vi "Periodic Tasks.vi"(8 "error in":errorcluster, 11 "RobotConfig":T3={"Motors"={"DriveRightPrimary"={"CAN Address"=3, "Invert"=FALSE, "InvertSensor"=FALSE, "Unit Conversion Factor"=0.0, "Brake Mode"=enum."Override to Brake", "Reverse Limt Switch Mode"=enum."Normally Closed", "Forward Limt Swith Mode"=enum."Normally Closed", "PWM Channel"=enum."Invalid", "Motor Controller Type"=enum."Talon SRX"}, "DriveRightSecondary"={"CAN Address"=2, "Invert"=FALSE, "InvertSensor"=FALSE, "Unit Conversion Factor"=0.0, "Brake Mode"=enum."Override to Brake", "Reverse Limt Switch Mode"=enum."Normally Closed", "Forward Limt Swith Mode"=enum."Normally Closed", "PWM Channel"=enum."Invalid", "Motor Controller Type"=enum."Talon SRX"}, "DriveLeftPrimary"={"CAN Address"=1, "Invert"=FALSE, "InvertSensor"=FALSE, "Unit Conversion Factor"=0.0, "Brake Mode"=enum."Override to Brake", "Reverse Limt Switch Mode"=enum."Normally Closed", "Forward Limt Swith Mode"=enum."Normally Closed", "PWM Channel"=enum."Invalid", "Motor Controller Type"=enum."Talon SRX"}, "DriveLeftSecondary"={"CAN Address"=4, "Invert"=FALSE, "InvertSensor"=FALSE, "Unit Conversion Factor"=0.0, "Brake Mode"=enum."Override to Brake", "Reverse Limt Switch Mode"=enum."Normally Closed", "Forward Limt Swith Mode"=enum."Normally Closed", "PWM Channel"=enum."Invalid", "Motor Controller Type"=enum."Talon SRX"}, "RearClimb"={"CAN Address"=8, "Invert"=FALSE, "InvertSensor"=FALSE, "Unit Conversion Factor"=0.0, "Brake Mode"=enum."Override to Brake", "Reverse Limt Switch Mode"=enum."Normally Closed", "Forward Limt Swith Mode"=enum."Normally Closed", "PWM Channel"=enum."Invalid", "Motor Controller Type"=enum."Talon SRX"}, "Front Climb"={"CAN Address"=7, "Invert"=FALSE, "InvertSensor"=FALSE, "Unit Conversion Factor"=0.0, "Brake Mode"=enum."Override to Brake", "Reverse Limt Switch Mode"=enum."Normally Closed", "Forward Limt Swith Mode"=enum."Normally Closed", "PWM Channel"=enum."Invalid", "Motor Controller Type"=enum."Talon SRX"}, "Climb Drive"={"CAN Address"=5, "Invert"=FALSE, "InvertSensor"=FALSE, "Unit Conversion Factor"=0.0, "Brake Mode"=enum."Override to Brake", "Reverse Limt Switch Mode"=enum."Normally Closed", "Forward Limt Swith Mode"=enum."Normally Closed", "PWM Channel"=enum."Invalid", "Motor Controller Type"=enum."Talon SRX"}, "Shoulder1"={"CAN Address"=6, "Invert"=FALSE, "InvertSensor"=FALSE, "Unit Conversion Factor"=0.0, "Brake Mode"=enum."Override to Brake", "Reverse Limt Switch Mode"=enum."Normally Closed", "Forward Limt Swith Mode"=enum."Normally Closed", "PWM Channel"=enum."Invalid", "Motor Controller Type"=enum."Talon SRX"}, "Shoulder2"={"CAN Address"=9, "Invert"=FALSE, "InvertSensor"=FALSE, "Unit Conversion Factor"=0.0, "Brake Mode"=enum."Override to Brake", "Reverse Limt Switch Mode"=enum."Normally Closed", "Forward Limt Swith Mode"=enum."Normally Closed", "PWM Channel"=enum."Invalid", "Motor Controller Type"=enum."Talon SRX"}, "Wrist"={"CAN Address"=10, "Invert"=FALSE, "InvertSensor"=FALSE, "Unit Conversion Factor"=0.0, "Brake Mode"=enum."Override to Brake", "Reverse Limt Switch Mode"=enum."Disabled", "Forward Limt Swith Mode"=enum."Disabled", "PWM Channel"=enum."Invalid", "Motor Controller Type"=enum."Talon SRX"}, "Extension"={"CAN Address"=11, "Invert"=FALSE, "InvertSensor"=FALSE, "Unit Conversion Factor"=0.0, "Brake Mode"=enum."Override to Brake", "Reverse Limt Switch Mode"=enum."Disabled", "Forward Limt Swith Mode"=enum."Disabled", "PWM Channel"=enum."Invalid", "Motor Controller Type"=enum."Talon SRX"}, "Intake1"={"CAN Address"=11, "Invert"=FALSE, "InvertSensor"=FALSE, "Unit Conversion Factor"=0.0, "Brake Mode"=enum."Override to Brake", "Reverse Limt Switch Mode"=enum."Disabled", "Forward Limt Swith Mode"=enum."Disabled", "PWM Channel"=enum."Invalid", "Motor Controller Type"=enum."Talon SRX"}, "Intake2"={"CAN Address"=11, "Invert"=FALSE, "InvertSensor"=FALSE, "Unit Conversion Factor"=0.0, "Brake Mode"=enum."Override to Brake", "Reverse Limt Switch Mode"=enum."Disabled", "Forward Limt Swith Mode"=enum."Disabled", "PWM Channel"=enum."Invalid", "Motor Controller Type"=enum."Talon SRX"}}, "Sensors"={"IMU"={"Yaw Axis"=enum."Z", "SPI Bus"=enum."SPI MXP", "AHRS Algorithm"=enum."Complementary", "Calibration Time (s)"=3.0, "Calibrate On Open"=TRUE}}, "PID"={"PIDParams"={"P"=0.0, "I"=0.0, "D"=0.0, "F"=0.0, "IZone"=0.0}}, "Solenoids"={" Shifter"={"SolenoidChannel"=enum."Solenoid 3", "Invert"=FALSE}, "Intake 1"={"SolenoidChannel"=enum."Solenoid 0", "Invert"=FALSE}, "Intake 2"={"SolenoidChannel"=enum."Solenoid 0", "Invert"=FALSE}, "Claw"={"Forward Channel"=enum."Solenoid 0", "Invert"=FALSE, "Reverse Channel"=enum."Solenoid 0"}}, "Enable Compressor"=TRUE}) -> ()   [LabVIEW 2018]
doc: "This VI runs in parallel to other tasks. It can contain as many user-defined periodic loops as you need. These can carry out PID or other sorts of timed response."
uses:
  DeepSpaceSrc/TypeDefs/ConfigComponents/Config_Robot.ctl
  ArgosLib/Config/ConfigComponents/TypeDefs/Config_Motor.ctl
  <vilib>/Rock Robotics/WPI/ThirdParty/Phoenix-LabVIEW/Motor Controller/Controls/CTRE_Phoenix_MotorControl_NeutralMode.ctl
  <vilib>/Rock Robotics/WPI/ThirdParty/Phoenix-LabVIEW/Motor Controller/Controls/CTRE_Phoenix_MotorControl_LimitSwitchNormal.ctl
  <vilib>/Rock Robotics/SystemInterfaces/DIO/FPGA_DIOPWMChannel.ctl
  ArgosLib/Config/ConfigComponents/TypeDefs/Config_MotorCtrlType.ctl
  ArgosLib/Config/ConfigComponents/TypeDefs/Config_IMU.ctl
  <vilib>/Rock Robotics/SystemInterfaces/spilib/spi_bus.ctl
  ArgosLib/Config/ConfigComponents/TypeDefs/Config_PIDParams.ctl
  ArgosLib/Config/ConfigComponents/TypeDefs/Config_SingleSolenoid.ctl
  <vilib>/Rock Robotics/WPI/Solenoid/WPI_SolenoidChannel.ctl
  ArgosLib/Config/ConfigComponents/TypeDefs/Config_DoubleSolenoid.ctl
  ArgosLib/Miscellaneous/TypeDefs/ArgoDriveJoystickMap.ctl
  ArgosLib/Miscellaneous/TypeDefs/LookUpTableParameters.ctl
  <vilib>/Rock Robotics/WPI/Solenoid/WPI_SolenoidValue.ctl
  <vilib>/Rock Robotics/WPI/Utilities/WPI_GetSetVariantRefNum.vi
  DeepSpaceSrc/Global_Var-RefNum/Joystick_Control.vi
  <vilib>/Rock Robotics/WPI/Solenoid/WPI_SolenoidSetEnum.vi
  ArgosLib/ArgosLib.lvlib
panel:
  in  "Argo Drive Joystick Map":T1={"Auto Speed"={"Look Up Table OUT"=[-1.0, 0.0, 0.0, 0.0, 1.0], "Look Up Table IN"=[-1.0, -0.1, 0.0, 0.1, 1.0]}, "Low Speed"={"Look Up Table OUT"=[-1.0, 0.0, 0.0, 0.0, 1.0], "Look Up Table IN"=[-1.0, -0.1, 0.0, 0.1, 1.0]}, "Auto Turning"={"Look Up Table OUT"=[-1.0, -0.1, 0.0, 0.1, 1.0], "Look Up Table IN"=[-1.0, -0.1, 0.0, 0.1, 1.0]}, "Low Turning"={"Look Up Table OUT"=[-1.0, 0.0, 0.0, 0.0, 1.0], "Look Up Table IN"=[-1.0, -0.1, 0.0, 0.1, 1.0]}, "High Speed"={"Look Up Table OUT"=[-1.0, 0.0, 0.0, 0.0, 1.0], "Look Up Table IN"=[-1.0, -0.1, 0.0, 0.1, 1.0]}, "High Turning"={"Look Up Table OUT"=[-1.0, 0.0, 0.0, 0.0, 1.0], "Look Up Table IN"=[-1.0, -0.1, 0.0, 0.1, 1.0]}}
  out "LED Loop Rate (Hz)":dbl
  out "Implement Loop Rate (Hz)":dbl
  out "Compressor Loop Rate (Hz)":dbl
  out "Drive Loop Rate (Hz)":dbl
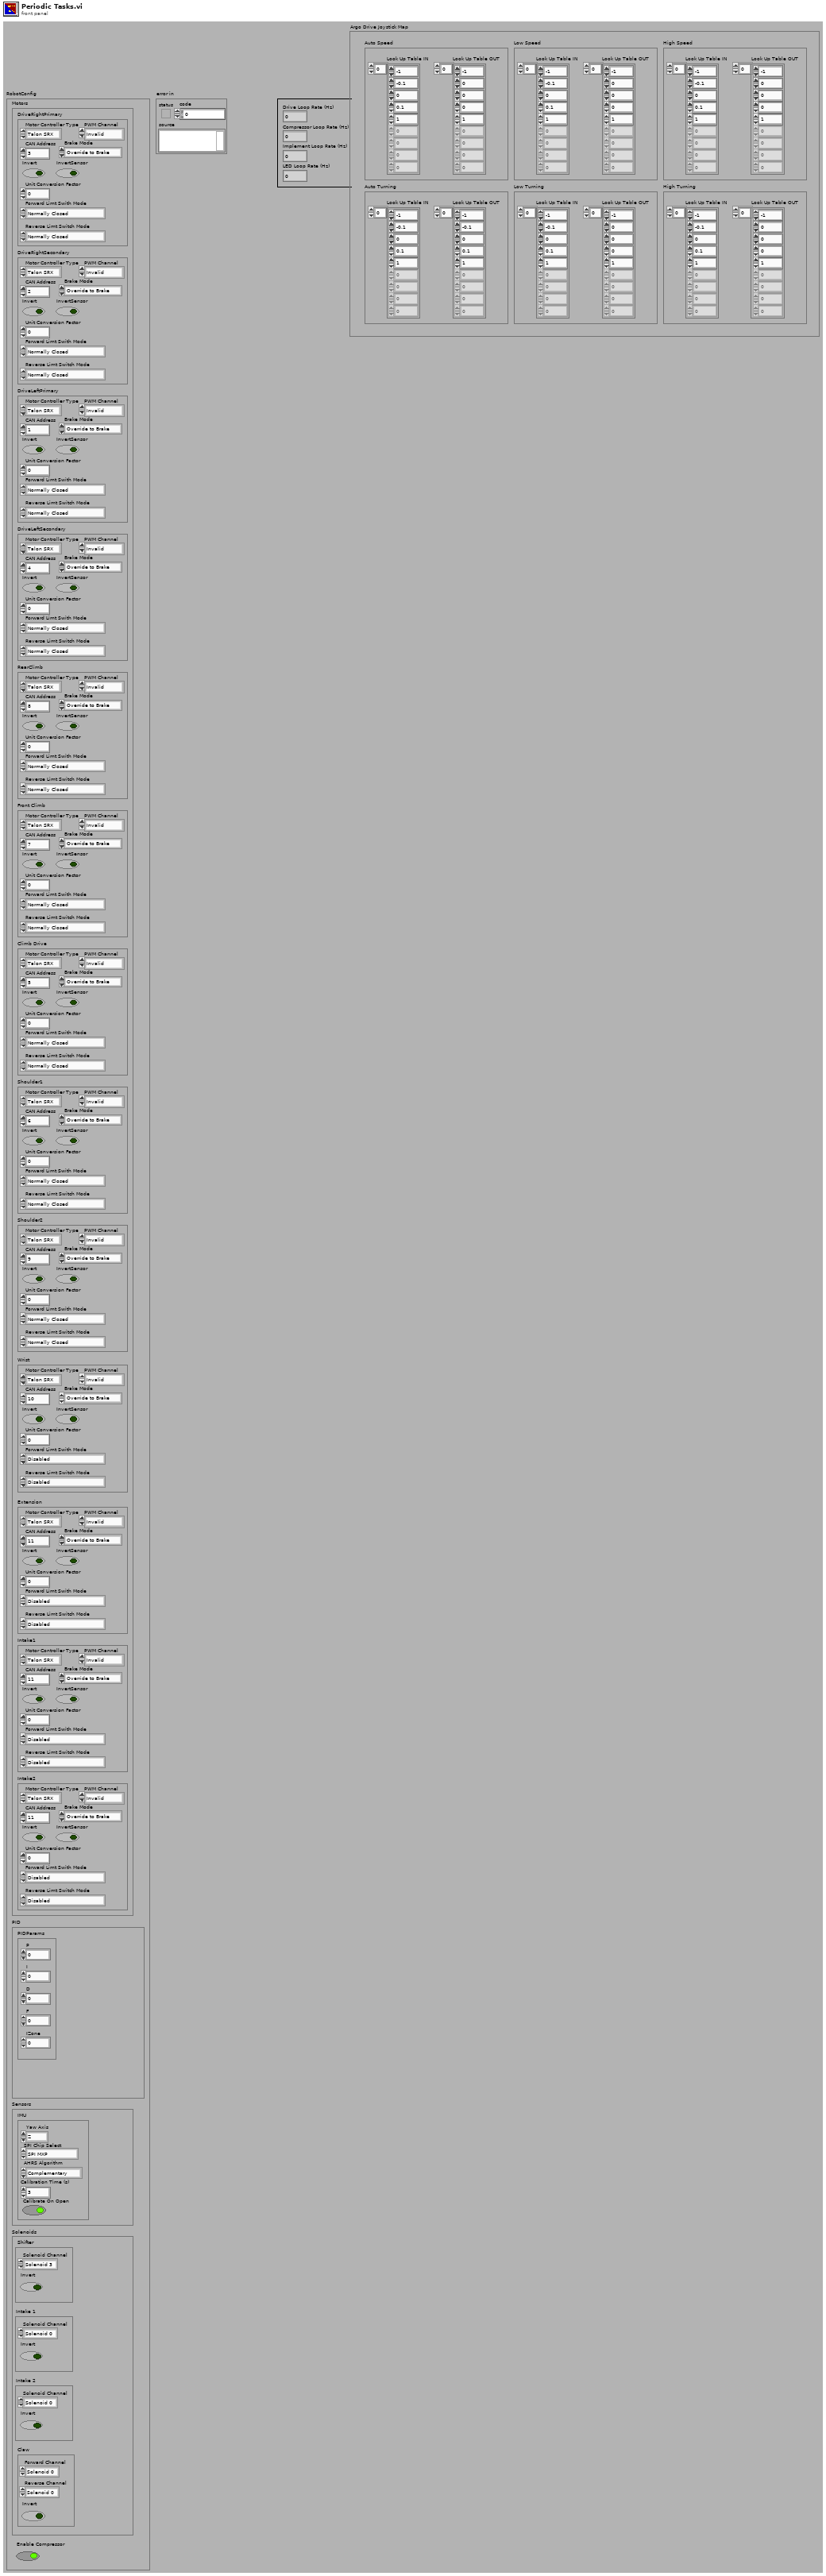
[diagram p1: front panel]
types:
  T1 = typedef "ArgosLib.lvlib/ArgoDriveJoystickMap.ctl" = cluster{"Auto Speed":T2, "Low Speed":T2, "Auto Turning":T2, "Low Turning":T2, "High Speed":T2, "High Turning":T2}
  T2 = typedef "ArgosLib.lvlib/LookUpTableParameters.ctl" = cluster{"Look Up Table OUT":dbl[], "Look Up Table IN":dbl[]}
  T3 = typedef "Config_Robot.ctl" = cluster{"Motors":cluster{"DriveRightPrimary":T4, "DriveRightSecondary":T4, "DriveLeftPrimary":T4, "DriveLeftSecondary":T4, "RearClimb":T4, "Front Climb":T4, "Climb Drive":T4, "Shoulder1":T4, "Shoulder2":T4, "Wrist":T4, "Extension":T4, "Intake1":T4, "Intake2":T4}, "Sensors":cluster{"IMU":T9}, "PID":cluster{"PIDParams":T11}, "Solenoids":cluster{" Shifter":T12, "Intake 1":T12, "Intake 2":T12, "Claw":T14}, "Enable Compressor":bool}
  T4 = typedef "ArgosLib.lvlib/Config_Motor.ctl" = cluster{"CAN Address":u8, "Invert":bool, "InvertSensor":bool, "Unit Conversion Factor":dbl, "Brake Mode":T5, "Reverse Limt Switch Mode":T6, "Forward Limt Swith Mode":T6, "PWM Channel":T7, "Motor Controller Type":T8}
  T5 = typedef "CTRE_Phoenix_MotorControl_NeutralMode.ctl" = enum8{"EEPROMSetting", "Override to Coast", "Override to Brake"}
  T6 = typedef "CTRE_Phoenix_MotorControl_LimitSwitchNormal.ctl" = enum16{"Normally Open", "Normally Closed", "Disabled"}
  T7 = typedef "FPGA_DIOPWMChannel.ctl" = enum8{"PWM 0", "PWM 1", "PWM 2", "PWM 3", "PWM 4", "PWM 5", "PWM 6", "PWM 7", "PWM 8", "PWM 9", "PWM MXP 0", "PWM MXP 1", "PWM MXP 2", "PWM MXP 3", "PWM MXP 4", "PWM MXP 5", "PWM MXP 6", "PWM MXP 7", "PWM MXP 8", "PWM MXP 9", "Invalid"}
  T8 = typedef "ArgosLib.lvlib/Config_MotorCtrlType.ctl" = enum16{"Disabled", "Talon SRX", "Talon SR"}
  T9 = typedef "ArgosLib.lvlib/Config_IMU.ctl" = cluster{"Yaw Axis":enum16{"X", "Y", "Z"}, "SPI Bus":T10, "AHRS Algorithm":enum16{"Complementary", "Madgwick"}, "Calibration Time (s)":dbl, "Calibrate On Open":bool}
  T10 = typedef "spi_bus.ctl" = enum16{"SPI On-Board, CS0", "SPI On-Board, CS1", "SPI On-Board, CS2", "SPI On-Board, CS3", "SPI MXP", "Invalid"}
  T11 = typedef "ArgosLib.lvlib/Config_PIDParams.ctl" = cluster{"P":dbl, "I":dbl, "D":dbl, "F":dbl, "IZone":dbl}
  T12 = typedef "ArgosLib.lvlib/Config_SingleSolenoid.ctl" = cluster{"SolenoidChannel":T13, "Invert":bool}
  T13 = typedef "WPI_SolenoidChannel.ctl" = enum8{"Solenoid 0", "Solenoid 1", "Solenoid 2", "Solenoid 3", "Solenoid 4", "Solenoid 5", "Solenoid 6", "Solenoid 7", "Invalid"}
  T14 = typedef "ArgosLib.lvlib/Config_DoubleSolenoid.ctl" = cluster{"Forward Channel":T13, "Invert":bool, "Reverse Channel":T13}
  T15 = typedef "RobotJoysticks.ctl" = cluster{"Driver Controller":T16, "Operator Controller":T16, "Manual Controller":T16}
  T16 = typedef "WPI_JoystickDevRef.ctl" = cluster{"Device":T17}
  T17 = typedef "WPI_JoystickDeviceEnum.ctl" = enum16{"USB 0", "USB 1", "USB 2", "USB 3", "USB 4", "USB 5"}
  T18 = typedef "WPI_RobotDriveDevRef.ctl" = cluster{"DevStatus":errorcluster, "Motors[]":T19[], "Square Inputs":bool, "Max Output":dbl}
  T19 = typedef "WPI_MotorControlDeviceRef.ctl" = cluster{"DeviceStatus":errorcluster, "Type":T20, "PWM":cluster{"PWM Channel":T7, "DeadBand":T21}, "CAN":cluster{"Device Number":u8, "SetOutput VI Ref":variant, "GetOutput VI Ref":variant, "Enable VI Ref":variant, "Disable VI Ref":variant, "Data":variant}, "Invert":bool, "DIO PWM":cluster{"PWM \"Enable\" Channel":T7, "DIOChannel":T22, "PWM Rate":dbl}}
  T20 = typedef "WPI_MotorControlType.ctl" = enum16{"PWM", "CAN", "DIO PWM"}
  T21 = typedef "WPI_PWMDeadband.ctl" = cluster{"Name":string, "maxPositivePwm":i32, "minPositivePwm":i32, "centerPwm":i32, "maxNegativePwm":i32, "minNegativePwm":i32, "angularRange":u16}
  T22 = typedef "FPGA_DIOChannel.ctl" = enum8{"DIO 0", "DIO 1", "DIO 2", "DIO 3", "DIO 4", "DIO 5", "DIO 6", "DIO 7", "DIO 8", "DIO 9", "DIO MXP 0", "DIO MXP 1", "DIO MXP 2", "DIO MXP 3", "DIO MXP 4", "DIO MXP 5", "DIO MXP 6", "DIO MXP 7", "DIO MXP 8", "DIO MXP 9", "DIO MXP 10", "DIO MXP 11", "DIO MXP 12", "DIO MXP 13", "DIO MXP 14", "DIO MXP 15", "SPI Port CS1", "SPI Port CS2", "SPI Port CS3", "SPI Port MISO", "SPI Port MOSI", "Invalid"}
  T23 = typedef "RobotMotors.ctl" = cluster{"DriveRightPrimary":T19, "DriveRightSecondary":T19, "DriveLeftPrimary":T19, "DriveLeftSecondary":T19, " RearClimb":T19, "FrontClimb":T19, "ClimbDrive":T19, "Shoulder2":T19, "Shoulder1 ":T19, "Wrist":T19, "Extension":T19, "Intake1":T19, "Intake2":T19}
  T24 = typedef "RobotPneumatics.ctl" = cluster{"Shifter":T25, "Compressor":T26, "Claw":T25, "Intake 1":T25, "Intake 2":T25}
  T25 = typedef "WPI_SolenoidDevRef.ctl" = cluster{"DevStatus":errorcluster, "Pneumatics Control Module":u8, "Forward Solenoid Channel":T13, "Reverse Solenoid Channel":T13}
  T26 = typedef "WPI_CompressorDevRef.ctl" = cluster{"DevStatus":errorcluster, "Pneumatics Control Module":u8}
  T27 = typedef "RobotSensors.ctl" = cluster{"DigitalIOConfig":T28}
  T28 = typedef "ArgosLib.lvlib/Config_DigitalIO.ctl" = cluster{"DIOChannel":T22, "Active Low":bool}
  T29 = cluster{"RobotConfig":T3, "Joysticks":T15, "RobotDriveDevRef":T18, "RobotMotorsOut":T23, "Pneumatics":T24, "Sensors":T27}
  T30 = typedef "WPI_SolenoidValue.ctl" = enum16{"Off", "On", "Forward", "Reverse"}
  T31 = typedef "JoystickControls.ctl" = cluster{"Drive":dbl, "Drive Turn ":dbl, "Unassigned_LX":dbl, "Unassigned_RY":dbl, "Claw Release":bool, "Back Intake Forward":dbl, "Front Intake Forward":dbl, "SP Low":bool, "SP Mid":bool, "SP High":bool, "Shift":bool, "Arm Go To Position":bool, "Unassigned_LJ":bool, "Unassigned_RJ":bool, "Swap_Back":bool, "Swap_Start":bool, "Unassigned_LY 2":dbl, "Unassigned_RX 2":dbl, "Unassigned_LX 2":dbl, "Unassigned_RY 2":dbl, "Claw Release 2":bool, "Back Intake REV":dbl, "Front Intake REV":dbl, "SP Low 2":bool, "SP Mid 2":bool, "SP High 2":bool, "Hatch/Cargo":bool, "Fwd/Rev":bool, "Unassigned_LJ 2":bool, "Unassigned_RJ 2":bool, "Swap_Back 2":bool, "Swap_Start 2":bool, "Unassigned_Up 2":bool, "Unassigned_Right 2":bool, "Arm Return":bool, "Unassigned_Left 2":bool, "Auto Climb":bool, " Unassigned_Right":bool, "Unassigned_Down":bool, "Unassigned_Left":bool, "Shoulder":dbl, "Unassigned_RX 3":dbl, "Unassigned_LX 3":dbl, "Arm Extend":dbl, "Climb Drive Reverse":bool, "Wrist CCW":dbl, "Wrist CW":dbl, "Rev Intake Extend":bool, "Fw Intake Extend":bool, "Climb Dr Forward":bool, "Intake Ingest ":bool, "Claw Release 3":bool, "Unassigned_LJ 3":bool, "Unassigned_RJ 3":bool, "Intake Puke":bool, "Unassigned Start 3":bool, "Climb F Up":bool, "Climb R Up":bool, "Climb F Down":bool, "Climb R Down":bool}
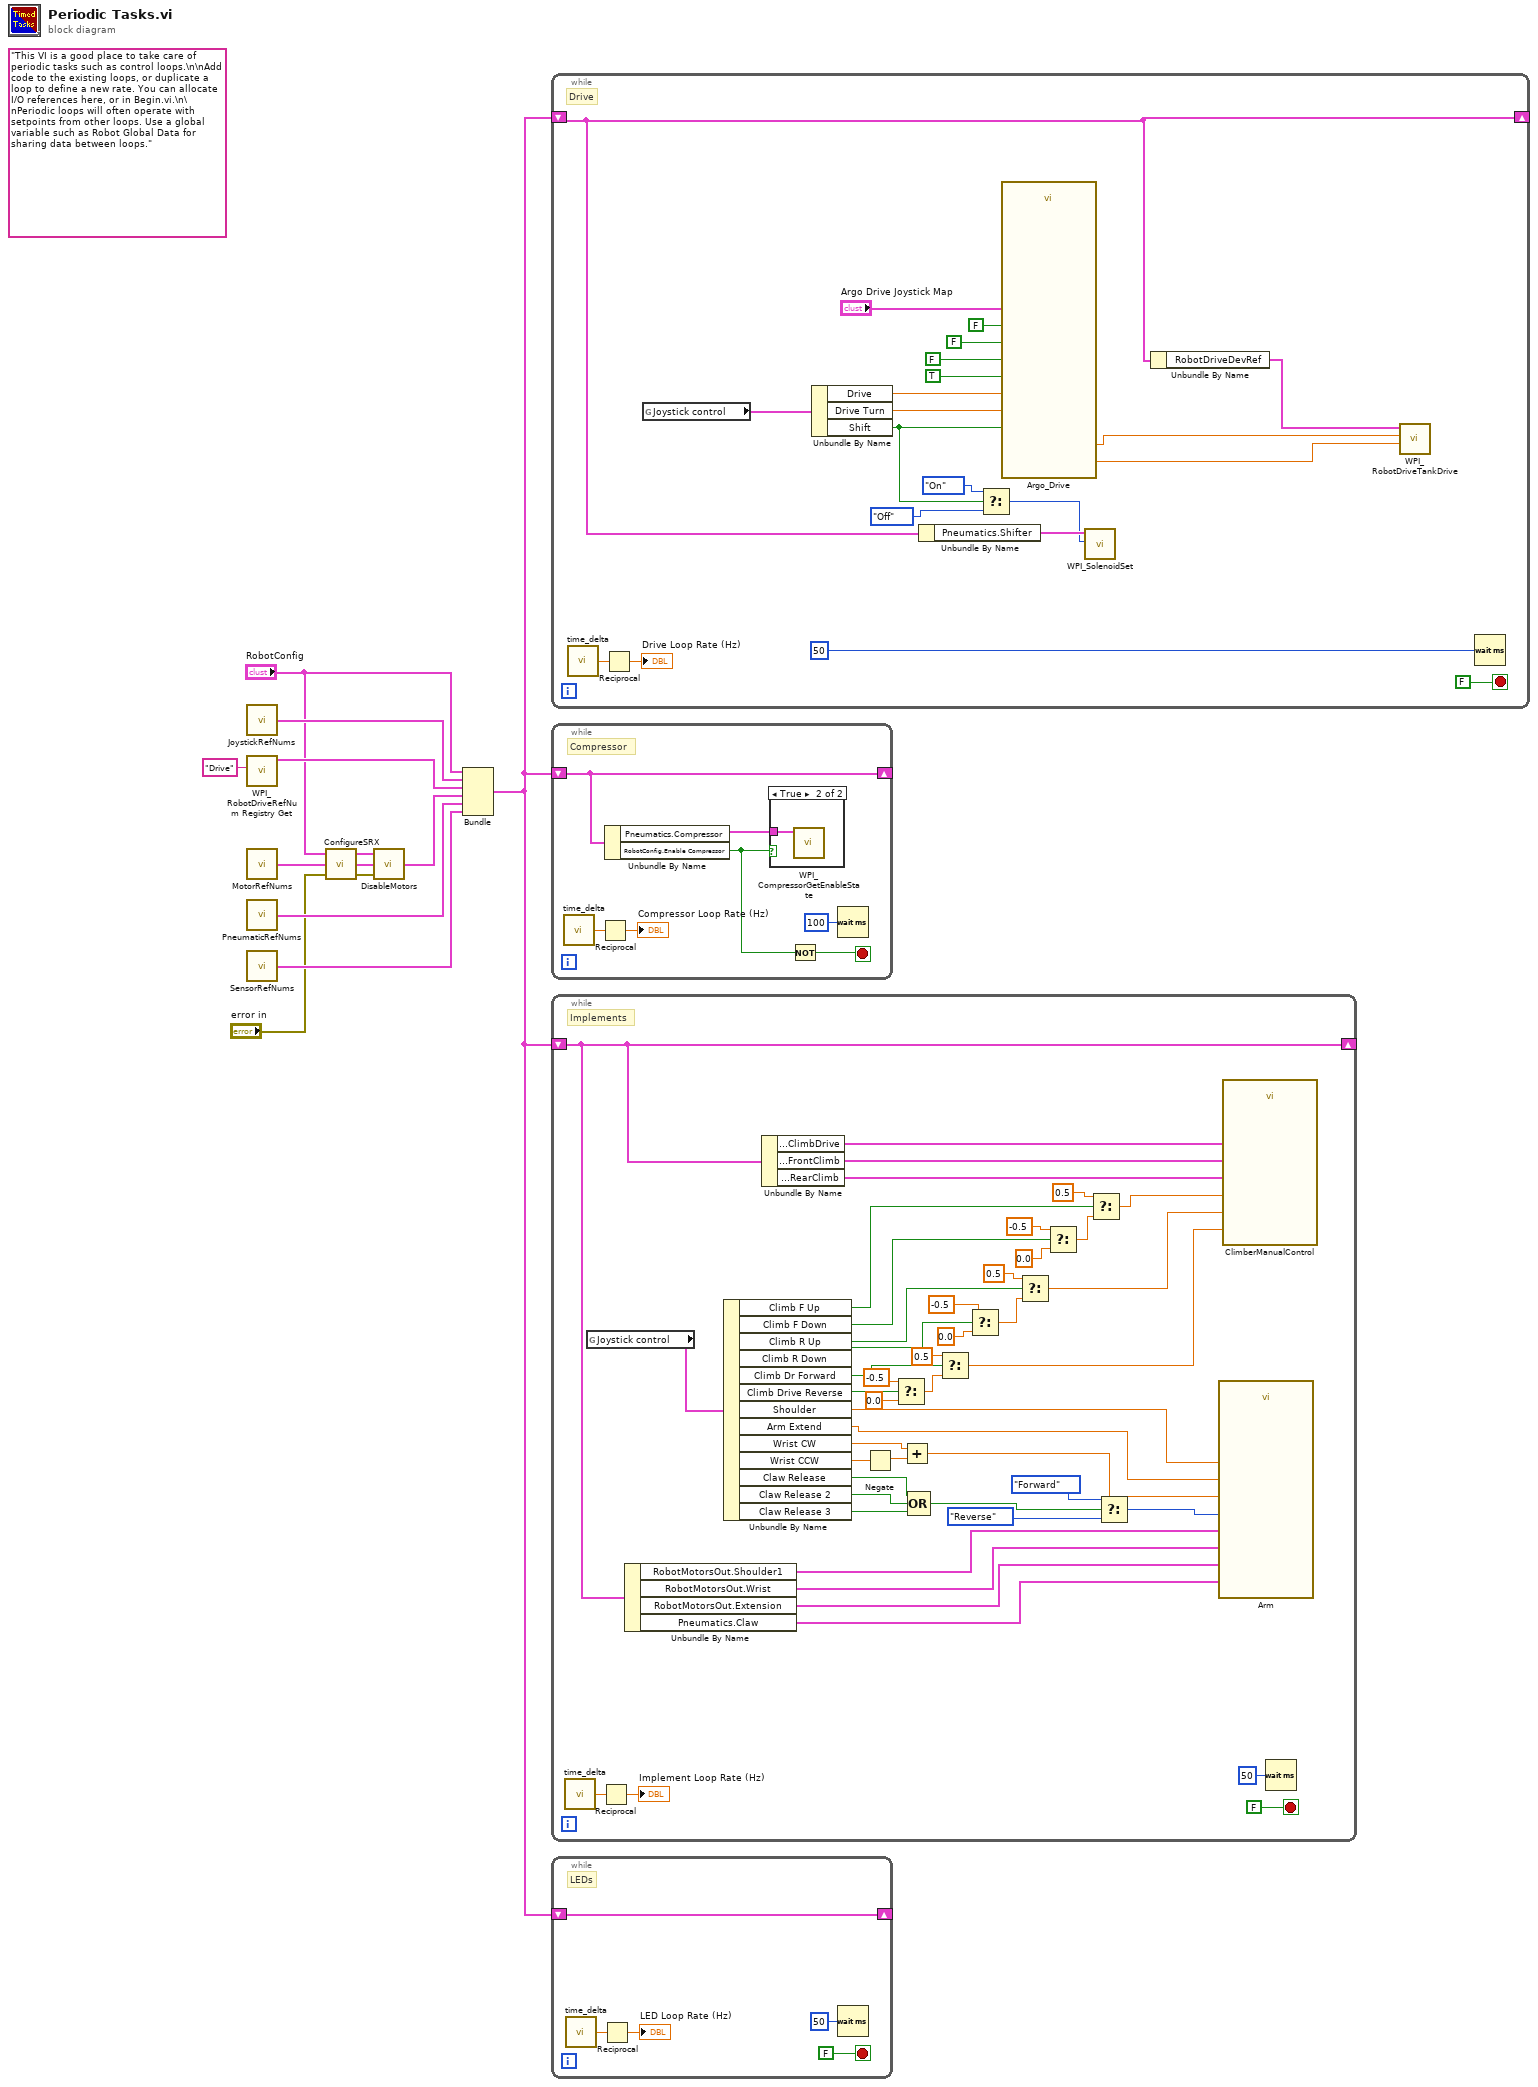
[diagram p0: block diagram]
diagram:
  (unwired) "This VI is a good place to take care of periodic tasks such as control loops.\n\nAdd code to the existing loops, or duplicate a loop to define a new rate. You can allocate I/O references here, or in Begin.vi.\n\nPeriodic loops will often operate with setpoints from other loops. Use a global variable such as Robot Global Data for sharing data between loops."
  n1 = call "JoystickRefNums.vi"() -> ("Joysticks"=w13:T15)  [unwired: 1 in]
  n2 = call <vilib>:"WPI_RobotDriveRefNum Registry Get.vi"("refnum name"="Drive") -> ("RobotDriveDevRef"=w12:T18)  [unwired: 9 in, 1 out]
  n3 = call "MotorRefNums.vi"() -> ("MotorRefNums"=w5:T23)  [unwired: 1 in]
  n4 = call "PneumaticRefNums.vi"() -> ("Pneumatics"=w11:T24)  [unwired: 1 in]
  n5 = call "SensorRefNums.vi"() -> ("Sensors"=w10:T27)  [unwired: 1 in]
  n6 = call "ConfigureSRX.vi"("error in"="error in", "RobotMotors"=w5, "RobotConfig"="RobotConfig") -> ("error out"=w9:errorcluster, "RobotMotorsOut"=w7:T23, "RobotConfigOut"=w8:T3)
  n7 = call "DisableMotors.vi"("error in"=w9, "RobotMotors"=w7, "RobotConfig"=w8) -> ("RobotMotorsOut"=w3:T23)  [unwired: 2 out]
  n8 = Bundle("RobotConfig"="RobotConfig", "Joysticks"=w13, "RobotDriveDevRef"=w12, "RobotMotorsOut"=w3, "Pneumatics"=w11, "Sensors"=w10) -> (w1:T29)  [unwired: 1 out]
  n9 = while {
    shift-right: [w19] -> _
    shift-left: w1 -> [w19]
    stop <- FALSE stop-if-true
    # "Drive"
    n10 = call "time_delta.vi"() -> ("dt (s)"=w32:dbl)  [unwired: 1 in]
    n11 = Reciprocal(x=w32) -> (1/x=→"Drive Loop Rate (Hz)":dbl)
    n12 = global read "Joystick_Control.vi" "Joystick control"() -> (w30:T31)
    n13 = Unbundle By Name(w30) -> ("Drive"=w28:dbl, "Drive Turn"=w29:dbl, "Shift"=w17:bool)
    n14 = Unbundle By Name(w19) -> ("Pneumatics.Shifter"=w18:T25)
    n15 = Select(t=WPI_SolenoidValue."On", s=w17, f=WPI_SolenoidValue."Off" ("Value")) -> (s? t:f=w15:T30)
    n16 = call "Argo_Drive.vi"("Speed_Main"=w28, "Argo Drive Joystick Map"="Argo Drive Joystick Map", "Backwards_Turning_Flip"=FALSE, "Turning_PID_Enable"=FALSE, "Turning_Main"=w29, "Auto_Enable"=FALSE, "High_Gear"=w17, "Quick_Turn"=TRUE) -> ("Left_Motor"=w22:dbl, "Right_Motor"=w21:dbl)  [unwired: 10 in]
    n17 = call-poly <vilib>:"WPI_SolenoidSet.vi"("Value"=w15, "SolenoidDevRef"=w18) -> ()  [unwired: 8 in, 2 out]
    n18 = Unbundle By Name(w19) -> ("RobotDriveDevRef"=w20:T18)
    n19 = call <vilib>:"WPI_RobotDriveTankDrive.vi"("Right axis value"=w21, "Left axis value"=w22, "RobotDriveDevRef"=w20) -> ()  [unwired: 6 in, 3 out]
    n20 = Wait (ms)(milliseconds to wait=u32 50) -> ()  [unwired: 1 out]
  }
  n21 = while {
    shift-right: [w38] -> _
    shift-left: w1 -> [w38]
    stop <- w37 stop-if-true
    # "Compressor"
    n22 = call "time_delta.vi"() -> ("dt (s)"=w39:dbl)  [unwired: 1 in]
    n23 = Reciprocal(x=w39) -> (1/x=→"Compressor Loop Rate (Hz)":dbl)
    n24 = Unbundle By Name(w38) -> ("Pneumatics.Compressor"=w35:T26, "RobotConfig.Enable Compressor"=w36:bool)
    n25 = case shown="True" w36 {
      tunnel: w35 -> [_ w42]
      frame False {
      }
      frame True {
        n26 = call <vilib>:"WPI_CompressorGetEnableState.vi"("CompressorDevRef"=w42) -> ()  [unwired: 7 in, 4 out]
      }
    }
    n27 = Not(x=w36) -> (.not. x?=w37:bool)
    n28 = Wait (ms)(milliseconds to wait=u32 100) -> ()  [unwired: 1 out]
  }
  n29 = while {
    shift-right: [w60] -> _
    shift-left: w1 -> [w60]
    stop <- FALSE stop-if-true
    # "Implements"
    n30 = call "time_delta.vi"() -> ("dt (s)"=w87:dbl)  [unwired: 1 in]
    n31 = global read "Joystick_Control.vi" "Joystick control"() -> (w85:T31)
    n32 = Reciprocal(x=w87) -> (1/x=→"Implement Loop Rate (Hz)":dbl)
    n33 = Unbundle By Name(w60) -> ("RobotMotorsOut.Shoulder1"=w59:T19, "RobotMotorsOut.Wrist"=w58:T19, "RobotMotorsOut.Extension"=w57:T19, "Pneumatics.Claw"=w56:T25)
    n34 = Unbundle By Name(w85) -> ("Climb F Up"=w76:bool, "Climb F Down"=w77:bool, "Climb R Up"=w78:bool, "Climb R Down"=w79:bool, "Climb Dr Forward"=w80:bool, "Climb Drive Reverse"=w81:bool, "Shoulder"=w47:dbl, "Arm Extend"=w48:dbl, "Wrist CW"=w44:dbl, "Wrist CCW"=w46:dbl, "Claw Release"=w55:bool, "Claw Release 2"=w54:bool, "Claw Release 3"=w53:bool)
    n35 = Unbundle By Name(w60) -> ("RobotMotorsOut.ClimbDrive"=w84:T19, "RobotMotorsOut.FrontClimb"=w83:T19, "RobotMotorsOut.RearClimb"=w82:T19)
    n36 = Negate(x=w46) -> (-x=w45:dbl)
    n37 = Select(t=-0.5, s=w81, f=0.0) -> (s? t:f=w75:dbl)
    n38 = Add(x=w44, y=w45) -> (x+y=w43:dbl)
    n39 = Compound Arithmetic op=OR(w55, w54, w53) -> (w52:bool)
    n40 = Select(t=0.5, s=w80, f=w75) -> (s? t:f=w61:dbl)
    n41 = Select(t=-0.5, s=w79, f=0.0) -> (s? t:f=w74:dbl)
    n42 = Select(t=0.5, s=w78, f=w74) -> (s? t:f=w62:dbl)
    n43 = Select(t=-0.5, s=w77, f=0.0) -> (s? t:f=w73:dbl)
    n44 = Select(t=0.5, s=w76, f=w73) -> (s? t:f=w63:dbl)
    n45 = Select(t=WPI_SolenoidValue."Forward" ("Claw Position"), s=w52, f=WPI_SolenoidValue."Reverse") -> (s? t:f=w49:T30)
    n46 = call "Arm.Vi"("ArmRotateDevRef"=w59, "ArmRotateOutput"=w47, "Claw Position"=w49, "ArmWristDevRef"=w58, "ArmExtendOutput"=w48, "ArmExtendDevRef"=w57, "ClawDevRef"=w56, "ArmWristOutput"=w43) -> ()  [unwired: 8 in]
    n47 = call "ClimberManualControl.vi"("RearDriveOutput"=w62, "FrontDriveOutput"=w63, "ClimbDriveOutput"=w61, "RearDriveDevRef"=w82, "FrontDriveDevRef"=w83, "ClimbDriveDevRef"=w84) -> ()  [unwired: 6 in]
    n48 = Wait (ms)(milliseconds to wait=u32 50) -> ()  [unwired: 1 out]
  }
  n49 = while {
    shift-right: [w92] -> _
    shift-left: w1 -> [w92]
    stop <- FALSE stop-if-true
    # "LEDs"
    n50 = call "time_delta.vi"() -> ("dt (s)"=w90:dbl)  [unwired: 1 in]
    n51 = Reciprocal(x=w90) -> (1/x=→"LED Loop Rate (Hz)":dbl)
    n52 = Wait (ms)(milliseconds to wait=u32 50) -> ()  [unwired: 1 out]
  }
